vi "NI_axisLabeltoBooleanCluster.vi"(11 "Offset Axes":T1[](array[typedef]) items=["Axis 1"=1, "Axis 2"=2, "Axis 3"=3, "Axis 4"=4, "Axis 5"=5, "Axis 6"=6, "Axis 7"=7, "Axis 8"=8, "Vector Space 1"=17, "Vector Space 2"=18, "Vector Space 3"=19, "Vector Space 4"=20]) -> (3 "Axis/VS Map (Disabled)":T2)   [LabVIEW 2022 SP3]
uses:
  <vilib>/Motion/FlexMotion/CustomControls/CustomControls.llb/Axis # (8 axes).flx
  <vilib>/Motion/FlexMotion/CustomControls/CustomControls.llb/AxisOrVectorSpace To Configure.flx
panel:
  # "Enable"
  # "Disable"
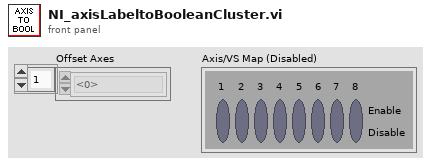
[diagram p1: front panel]
types:
  T1 = typedef "AxisOrVectorSpace To Configure.flx" = u16
  T2 = typedef "Axis # (8 axes).flx" = cluster{"1":bool, "2":bool, "3":bool, "4":bool, "5":bool, "6":bool, "7":bool, "8":bool}
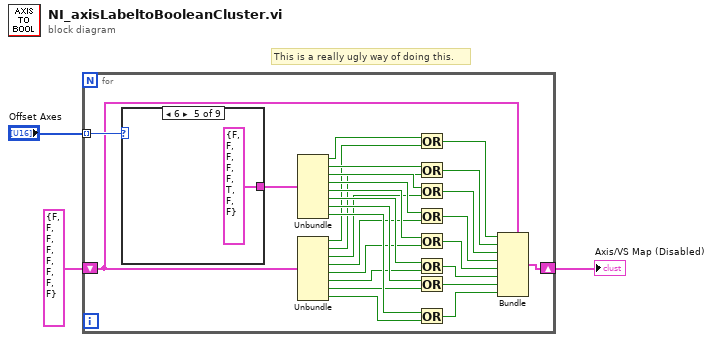
[diagram p0: block diagram]
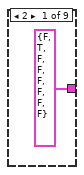
[diagram p2: hidden frame]
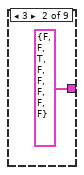
[diagram p3: hidden frame]
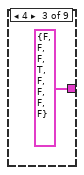
[diagram p4: hidden frame]
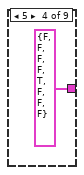
[diagram p5: hidden frame]
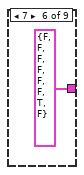
[diagram p6: hidden frame]
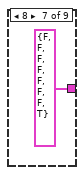
[diagram p7: hidden frame]
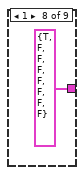
[diagram p8: hidden frame]
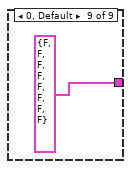
[diagram p9: hidden frame]
diagram:
  # "This is a really ugly way of doing this."
  n1 = for {
    shift-right: [w31] -> w3
    shift-left: T2 {"1"=FALSE, "2"=FALSE, "3"=FALSE, "4"=FALSE, "5"=FALSE, "6"=FALSE, "7"=FALSE, "8"=FALSE} ("Axis/VS Map (Disabled)") -> [w4]
    tunnel: "Offset Axes" -> [w6] mode=indexing
    n2 = case shown="6" w6 {
      tunnel: [T2 {"1"=FALSE, "2"=TRUE, "3"=FALSE, "4"=FALSE, "5"=FALSE, "6"=FALSE, "7"=FALSE, "8"=FALSE} ("Axis/VS Map (Disabled)") T2 {"1"=FALSE, "2"=FALSE, "3"=TRUE, "4"=FALSE, "5"=FALSE, "6"=FALSE, "7"=FALSE, "8"=FALSE} ("Axis/VS Map (Disabled)") T2 {"1"=FALSE, "2"=FALSE, "3"=FALSE, "4"=TRUE, "5"=FALSE, "6"=FALSE, "7"=FALSE, "8"=FALSE} ("Axis/VS Map (Disabled)") T2 {"1"=FALSE, "2"=FALSE, "3"=FALSE, "4"=FALSE, "5"=TRUE, "6"=FALSE, "7"=FALSE, "8"=FALSE} ("Axis/VS Map (Disabled)") T2 {"1"=FALSE, "2"=FALSE, "3"=FALSE, "4"=FALSE, "5"=FALSE, "6"=TRUE, "7"=FALSE, "8"=FALSE} ("Axis/VS Map (Disabled)") T2 {"1"=FALSE, "2"=FALSE, "3"=FALSE, "4"=FALSE, "5"=FALSE, "6"=FALSE, "7"=TRUE, "8"=FALSE} ("Axis/VS Map (Disabled)") T2 {"1"=FALSE, "2"=FALSE, "3"=FALSE, "4"=FALSE, "5"=FALSE, "6"=FALSE, "7"=FALSE, "8"=TRUE} ("Axis/VS Map (Disabled)") T2 {"1"=TRUE, "2"=FALSE, "3"=FALSE, "4"=FALSE, "5"=FALSE, "6"=FALSE, "7"=FALSE, "8"=FALSE} ("Axis/VS Map (Disabled)") T2 {"1"=FALSE, "2"=FALSE, "3"=FALSE, "4"=FALSE, "5"=FALSE, "6"=FALSE, "7"=FALSE, "8"=FALSE} ("Axis/VS Map (Disabled)")] -> w5
      frame 2 {
      }
      frame 3 {
      }
      frame 4 {
      }
      frame 5 {
      }
      frame 6 {
      }
      frame 7 {
      }
      frame 8 {
      }
      frame 1 {
      }
      frame 0, Default {
      }
    }
    n3 = Unbundle(w5) -> ("1"=w22:bool, "2"=w21:bool, "3"=w20:bool, "4"=w19:bool, "5"=w18:bool, "6"=w17:bool, "7"=w16:bool, "8"=w15:bool)
    n4 = Unbundle(w4) -> ("1"=w7:bool, "2"=w8:bool, "3"=w9:bool, "4"=w10:bool, "5"=w11:bool, "6"=w12:bool, "7"=w13:bool, "8"=w14:bool)
    n5 = Or(x=w22, y=w7) -> (x .or. y?=w30:bool)
    n6 = Or(x=w21, y=w8) -> (x .or. y?=w23:bool)
    n7 = Or(x=w20, y=w9) -> (x .or. y?=w24:bool)
    n8 = Or(x=w19, y=w10) -> (x .or. y?=w25:bool)
    n9 = Or(x=w18, y=w11) -> (x .or. y?=w26:bool)
    n10 = Or(x=w17, y=w12) -> (x .or. y?=w27:bool)
    n11 = Or(x=w16, y=w13) -> (x .or. y?=w28:bool)
    n12 = Or(x=w15, y=w14) -> (x .or. y?=w29:bool)
    n13 = Bundle(cluster=w4, "1"=w30, "2"=w23, "3"=w24, "4"=w25, "5"=w26, "6"=w27, "7"=w28, "8"=w29) -> (w31:T2)
  }
  "Axis/VS Map (Disabled)" <- w3
